vi "Set Name.vi"(8 "error in (no error)":errorcluster, 10 "Name":string, 11 "User BluelinesRedlines in":refnum<class "User BluelinesRedlines.lvclass">) -> (0 "error out":errorcluster, 3 "User BluelinesRedlines out":refnum<class "User BluelinesRedlines.lvclass">)   [LabVIEW 2020, in "VolatusGUIElements.lvlib" / "User BluelinesRedlines.lvclass"]
uses:
  User BluelinesRedlines.lvclass
  User BluelinesRedlines.lvclass/User BluelinesRedlines.ctl
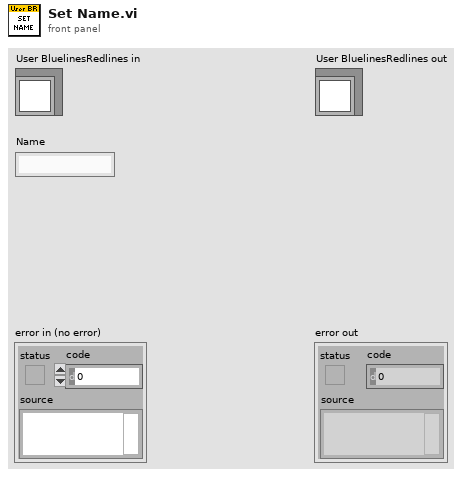
[diagram p1: front panel]
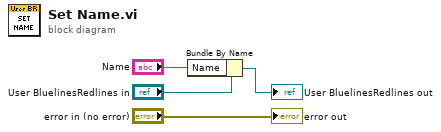
[diagram p0: block diagram]
diagram:
  n1 = Bundle By Name(cluster="User BluelinesRedlines in", "Name"="Name") -> (→"User BluelinesRedlines out":refnum<class "User BluelinesRedlines.lvclass">)
  "error out" <- "error in (no error)"
